vi "PH_Waveplate-GUI_6P.ProcCases.vi"(0 "i ref in":refnum<vi>, 1 "selector":string, 2 "data":i8[](array[numeric]), 3 "call cluster":T1={"Object"="", "Selector"="", "CallType"=enum."synchronous", "Async Object"="", "Async Selector"="", "Data Descriptor"="", "Data"=[], "Error #"=0, "Expire"=0}, 5 "error in":errorcluster) -> (14 "i ref out":refnum<vi>, 17 "answer cluster":T1={"Object"="", "Selector"="", "CallType"=enum."synchronous", "Async Object"="", "Async Selector"="", "Data Descriptor"="", "Data"=[], "Error #"=0, "Expire"=0}, 19 "error out":errorcluster)   [LabVIEW 2014, in "PH_Waveplate-GUI_6P.lvlib"]
doc: "This method is called by a process from within the default case in the event loop. The methods of a class that are linked to events will be called from THIS method. Add your code here."
uses:
  PH_Waveplate-GUI_6P.lvlib
  CSCore/CSSystem/CoreDefs/CoreDefs.call_type.ctl
  CSCore/BaseProcess/BaseProcess.descriptor string definition.ctl
  CSCore/CSSystem/CoreDefs/CoreDefs.rawDataType.ctl
  CSCore/CSSystem/CoreLib/CoreLib.string 2 byte array.vi
  CSCore/BaseProcess/BaseProcess.lvlib
  CSCore/CSSystem/CoreLib/CoreLib.lvlib
  PH_AxisGUI_BaseClass/PH_AxisGUI_BaseClass.lvlib
  PH_Stepmotor_BaseClass/PH_Stepmotor_BaseClass.lvlib
  CSCore/CAEObj/CAEObj.lvlib
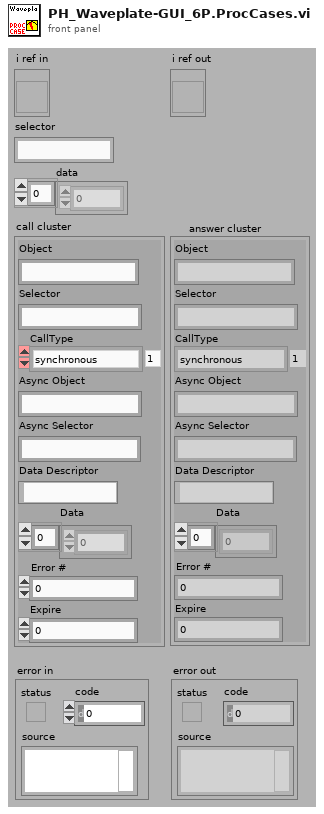
[diagram p1: front panel]
types:
  T1 = typedef "CoreDefs.call_type.ctl" = cluster{"Object":string, "Selector":string, "CallType":enum16{"simple", "synchronous", "asynchronous"}, "Async Object":string, "Async Selector":string, "Data Descriptor":T2, "Data":T3, "Error #":i32, "Expire":u32}
  T2 = typedef "BaseProcess.lvlib/BaseProcess.descriptor string definition.ctl" = string
  T3 = typedef "CoreDefs.rawDataType.ctl" = i8[]
  T4 = typedef "PH_Stepmotor_BaseClass.lvlib/PH_Stepmotor_BaseClass.Axis Settings.ctl" = cluster{"Sign change":bool, "Width":dbl, "Calibration":dbl, "Unit":string, "Motor Type":T5, "Unit Width":string, "Unit CF":string}
  T5 = typedef "PH_Stepmotor_BaseClass.lvlib/PH_Stepmotor_BaseClass.Motor Type.ctl" = enum16{"Unspecific", "OWIS 49.120.2633", "OWIS 49.060.1033", "OWIS 43.040.2558", "Diamond Motion 2200 series", "OWIS 49.120.266B.MV6", "Calorimeter", "Linear Stage 1", "MICOS VT-80", "MICOS VT-80 S", "Standa Rotstage nt0.95A", "PUF RA 320.200", "PUF RA 800.200", "PUF RA 800.400", "PUF RA 400.50", "1324.nn.800.50", "1324.n9c.800.50", "1324.nn.320.200", "1324.nn.400.200", "1324.nn.800.200", "1324.nn.400.50", "1324.8c9c.800.50", "1324.8c9c.400.200"}
  T6 = typedef "PH_Stepmotor_BaseClass.lvlib/PH_Stepmotor_BaseClass.Axis Information.ctl" = cluster{"Scaled Position":dbl, "Activity":T7}
  T7 = typedef "PH_Stepmotor_BaseClass.lvlib/PH_Stepmotor_BaseClass.Axis Activity.ctl" = enum16{"No Information", "stopped", "running", "Failure", "Alarm", "stopped at backward ES", "stopped at foreward ES"}
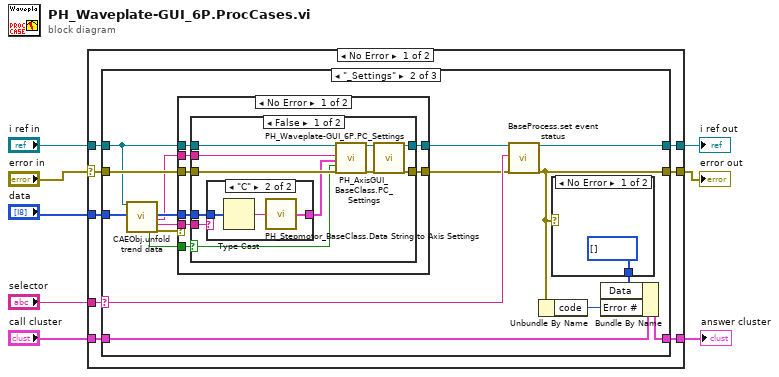
[diagram p0: block diagram]
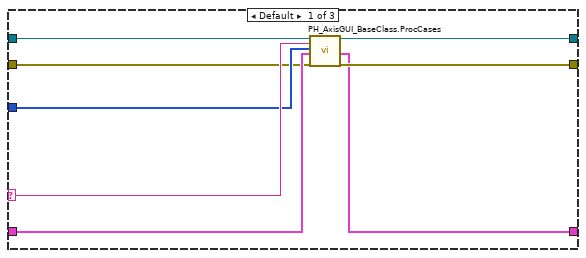
[diagram p2: hidden frame]
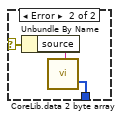
[diagram p6: hidden frame]
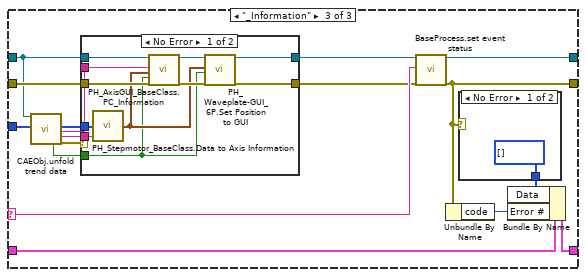
[diagram p7: hidden frame]
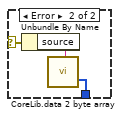
[diagram p9: hidden frame]
diagram:
  n1 = case shown="No Error" "error in" {
    selector: "error in" -> [w9 w107]
    tunnel: "selector" -> [w16 _]
    tunnel: [w15 w106] -> w7
    tunnel: "call cluster" -> [w14 w106]
    tunnel: "i ref in" -> [w13 w108]
    tunnel: [w12 w108] -> w4
    tunnel: [w11 w107] -> w3
    tunnel: "data" -> [w10 _]
    frame No Error {
      n2 = case shown="\"_Settings\"" w16 {
        selector: w16 -> [w20 w35 w85]
        tunnel: w13 -> [w19 w27 w74]
        tunnel: [w24 w38 w84] -> w12
        tunnel: w14 -> [w21 w40 w87]
        tunnel: [w22 w36 w82] -> w15
        tunnel: w9 -> [w17 w34 w81]
        tunnel: [w23 w39 w86] -> w11
        tunnel: w10 -> [w18 w30 w80]
        frame Default {
          n3 = call "PH_AxisGUI_BaseClass.ProcCases.vi"("i ref in"=w19, "selector"=w20, "data"=w18, "call cluster"=w21, "error in"=w17) -> ("i ref out"=w24:refnum<vi>, "answer cluster"=w22:T1, "error out"=w23:errorcluster)  [unwired: 12 in]
        }
        frame "_Settings" {
          n4 = call "CAEObj.unfold trend data.vi"("i ref in"=w27, "raw trend data"=w30) -> ("no link"=w28:bool, "data"=w31:i8[], "serviceName"=w25:string, "typeDescriptor"=w26:string, "error out"=w29:errorcluster)  [unwired: 9 in, 4 out]
          n5 = case shown="No Error" w29 {
            tunnel: w31 -> [w44 _]
            tunnel: w27 -> [w48 w67]
            tunnel: [w47 w67] -> w33
            tunnel: w34 -> [w49 w66]
            tunnel: [w46 w66] -> w32
            tunnel: w28 -> [w45 _]
            tunnel: w26 -> [w43 _]
            tunnel: w25 -> [w42 _]
            frame No Error {
              n6 = case "NO LINK?" shown="False" w45 {
                selector: w45 -> [w54 _]
                tunnel: w49 -> [w59 w65]
                tunnel: w48 -> [w60 w64]
                tunnel: [w51 w64] -> w47
                tunnel: [w50 w65] -> w46
                tunnel: w43 -> [w57 _]
                tunnel: w44 -> [w58 _]
                tunnel: w42 -> [w56 _]
                frame False {
                  n7 = case shown="\"C\"" w57 {
                    tunnel: [_ w61] -> w55
                    tunnel: w58 -> [_ w63]
                    frame Default {
                    }
                    frame "C" {
                      n8 = Type Cast(x=w63) -> (*(type *) &x=w62:string)  [unwired: 1 in]
                      n9 = call "PH_Stepmotor_BaseClass.Data String to Axis Settings.vi"("Data String"=w62) -> ("Axis Settings"=w61:T4)  [unwired: 1 out]
                    }
                  }
                  n10 = call "PH_AxisGUI_BaseClass.PC_Settings.vi"("i ref in"=w60, "Service Name"=w56, "Axis Settings"=w55, "No Link?"=w54, "error in"=w59) -> ("i ref out"=w52:refnum<vi>, "error"=w53:errorcluster)  [unwired: 12 in, 1 out]
                  n11 = call "PH_Waveplate-GUI_6P.PC_Settings.vi"("i ref in"=w52, "error in"=w53) -> ("i ref out"=w51:refnum<vi>, "error out"=w50:errorcluster)  [unwired: 16 in]
                }
                frame True {
                }
              }
            }
            frame Error {
            }
          }
          n12 = call "BaseProcess.set event status.vi"("i ref in"=w33, "EventStatus"=w35, "error in (no error)"=w32) -> ("i ref out"=w38:refnum<vi>, "error out"=w39:errorcluster)  [unwired: 14 in, 1 out]
          n13 = Unbundle By Name(w39) -> ("code"=w41:i32)
          n14 = case shown="No Error" w39 {
            selector: w39 -> [_ w71]
            tunnel: [T3 [] ("byteArray out") w69] -> w37
            frame No Error {
            }
            frame Error {
              n15 = Unbundle By Name(w71) -> ("source"=w70:string)
              n16 = call-poly "CoreLib.data 2 byte array.vi"("string"=w70) -> ("byteArray out"=w69:T3)  [unwired: 18 in]
            }
          }
          n17 = Bundle By Name(cluster=w40, "Data"=w37, "Error #"=w41) -> (w36:T1)
        }
        frame "_Information" {
          n18 = call "CAEObj.unfold trend data.vi"("i ref in"=w74, "raw trend data"=w80) -> ("no link"=w77:bool, "data"=w79:i8[], "serviceName"=w78:string, "typeDescriptor"=w75:string, "error out"=w76:errorcluster)  [unwired: 9 in, 4 out]
          n19 = case shown="No Error" w76 {
            tunnel: w79 -> [w98 _]
            tunnel: w74 -> [w96 w101]
            tunnel: [w90 w101] -> w73
            tunnel: w81 -> [w95 w100]
            tunnel: w77 -> [w91 _]
            tunnel: w75 -> [w97 _]
            tunnel: w78 -> [w99 _]
            tunnel: [w89 w100] -> w72
            frame No Error {
              n20 = call "PH_Stepmotor_BaseClass.Data to Axis Information.vi"("data"=w98, "Type Descriptor"=w97) -> ("Axis Information"=w92:T6)
              n21 = call "PH_AxisGUI_BaseClass.PC_Information.vi"("i ref in"=w96, "Service Name"=w99, "Axis Information"=w92, "no link"=w91, "error in"=w95) -> ("i ref out"=w94:refnum<vi>, "error out"=w93:errorcluster)  [unwired: 12 in, 1 out]
              n22 = call "PH_Waveplate-GUI_6P.Set Position to GUI.vi"("i ref in"=w94, "Axis Information"=w92, "no link"=w91, "error in"=w93) -> ("i ref out"=w90:refnum<vi>, "error out"=w89:errorcluster)  [unwired: 14 in]
            }
            frame Error {
            }
          }
          n23 = call "BaseProcess.set event status.vi"("i ref in"=w73, "EventStatus"=w85, "error in (no error)"=w72) -> ("i ref out"=w84:refnum<vi>, "error out"=w86:errorcluster)  [unwired: 14 in, 1 out]
          n24 = Unbundle By Name(w86) -> ("code"=w88:i32)
          n25 = case shown="No Error" w86 {
            selector: w86 -> [_ w105]
            tunnel: [T3 [] ("byteArray out") w103] -> w83
            frame No Error {
            }
            frame Error {
              n26 = Unbundle By Name(w105) -> ("source"=w104:string)
              n27 = call-poly "CoreLib.data 2 byte array.vi"("string"=w104) -> ("byteArray out"=w103:T3)  [unwired: 18 in]
            }
          }
          n28 = Bundle By Name(cluster=w87, "Data"=w83, "Error #"=w88) -> (w82:T1)
        }
      }
    }
    frame Error {
    }
  }
  "answer cluster" <- w7
  "i ref out" <- w4
  "error out" <- w3
